vi "file.jpg.Write.vi"(4 "Max Value":i32=97 min=1 max=65535, 6 "Min Value":i32=3 min=0 max=65535, 7 "name":string, 8 "error in":errorcluster, 10 "u16 pixmap":u16[][](array[numeric]), 11 "path":path) -> (0 "error out":errorcluster)   [LabVIEW 2020]
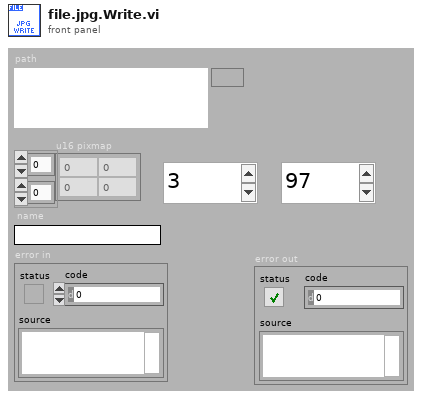
[diagram p1: front panel]
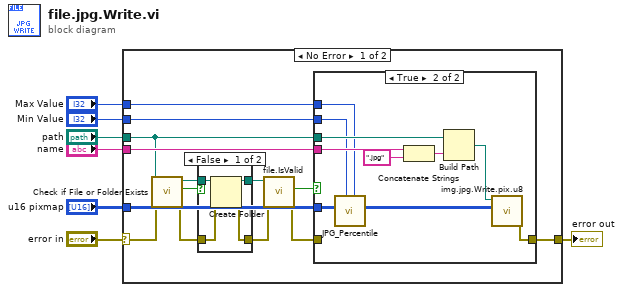
[diagram p0: block diagram]
diagram:
  n1 = case shown="No Error" "error in" {
    selector: "error in" -> [w19 w39]
    tunnel: "path" -> [w10 _]
    tunnel: "u16 pixmap" -> [w21 _]
    tunnel: [w20 w39] -> w4
    tunnel: "name" -> [w11 _]
    tunnel: "Max Value" -> [w9 _]
    tunnel: "Min Value" -> [w8 _]
    frame No Error {
      n2 = call <vilib>:"Check if File or Folder Exists.vi"("error in (no error)"=w19, "path"=w10) -> ("error out"=w17:errorcluster, "file or folder exists?"=w15:bool, "dup path"=w14:path)  [unwired: 7 in]
      n3 = case shown="False" w15 {
        tunnel: w14 -> [w36 w37]
        tunnel: w17 -> [w35 w38]
        tunnel: [w34 w38] -> w16
        tunnel: [w33 w37] -> w13
        frame False {
          n4 = Create Folder(path (use dialog)=w36, error in=w35) -> (created path=w33:path, error out=w34:errorcluster)  [unwired: 1 in, 1 out]
        }
        frame True {
        }
      }
      n5 = call "file.IsValid.vi"("error in (no error)"=w16, "path"=w13) -> ("error out"=w18:errorcluster, "valid file/folder?"=w12:bool)  [unwired: 7 in, 1 out]
      n6 = case shown="True" w12 {
        tunnel: w21 -> [_ w26]
        tunnel: [w22 w32] -> w20
        tunnel: w18 -> [w22 _]
        tunnel: w10 -> [_ w27]
        tunnel: w11 -> [_ w28]
        tunnel: w9 -> [_ w24]
        tunnel: w8 -> [_ w23]
        frame False {
        }
        frame True {
          n7 = call "JPG_Percentile.vi"("max"=w24, "min"=w23, "u16 pixmap 3"=w26) -> ("unsigned 8bit integer"=w25:u8[][])  [unwired: 8 in]
          n8 = Concatenate Strings(w28, ".jpg" ("string")) -> (w30:string)
          n9 = Build Path(base path=w27, name or relative path=w30) -> (appended path=w29:path)
          n10 = call "img.jpg.Write.pix.u8.vi"("pix.u8"=w25, "path"=w29) -> ("error out"=w32:errorcluster)  [unwired: 9 in]
        }
      }
    }
    frame Error {
    }
  }
  "error out" <- w4
